vi "labHolo_path.vi"(2 "sub folder or file (path)  [ignored if str is not empty]":path, 3 "sub folder or file (str)":string) -> (0 "Exists?":bool, 1 "labHolo path":path)   [LabVIEW 2022 SP3]
panel:
  out "sub folder names":string[](array[string])
  out "sub filenames":string[](array[string])
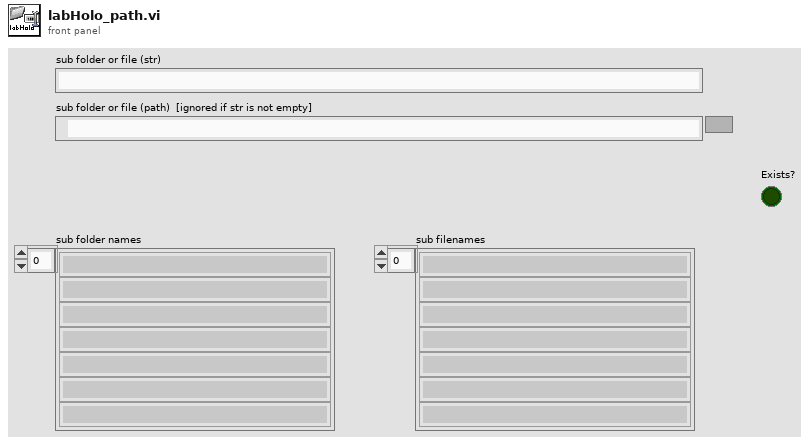
[diagram p1: front panel]
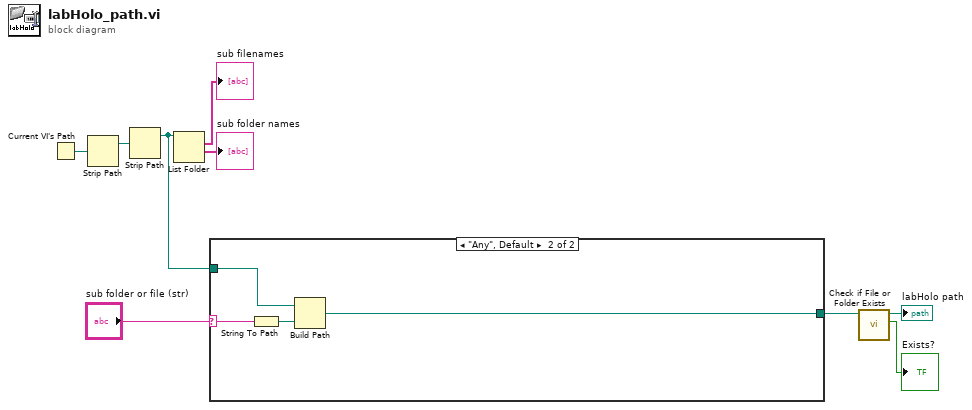
[diagram p0: block diagram]
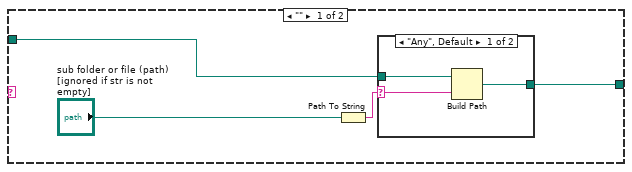
[diagram p2: hidden frame]
diagram:
  n1 = Current VI's Path() -> (path=w9:path)
  n2 = Strip Path(path=w9) -> (stripped path=w8:path)  [unwired: 1 out]
  n3 = Strip Path(path=w8) -> (stripped path=w4:path)  [unwired: 1 out]
  n4 = List Folder(path=w4) -> (filenames=→"sub filenames":string[], folder names=→"sub folder names":string[])  [unwired: 3 in, 2 out]
  n5 = case shown="\"Any\", Default" "sub folder or file (str)" {
    selector: "sub folder or file (str)" -> [_ w21]
    tunnel: w4 -> [w13 w19]
    tunnel: [w10 w20] -> w2
    frame "" {
      n6 = Path To String(path="sub folder or file (path)  [ignored if str is not empty]") -> (string=w11:string)
      n7 = case shown="\"Any\", Default" w11 {
        selector: w11 -> [w16 _]
        tunnel: w13 -> [w15 w17]
        tunnel: [w14 w17] -> w10
        frame "Any", Default {
          n8 = Build Path(base path=w15, name or relative path=w16) -> (appended path=w14:path)
        }
        frame "" {
        }
      }
    }
    frame "Any", Default {
      n9 = String To Path(string=w21) -> (path=w18:path)
      n10 = Build Path(base path=w19, name or relative path=w18) -> (appended path=w20:path)
    }
  }
  n11 = call <vilib>:"Check if File or Folder Exists.vi"("path"=w2) -> ("file or folder exists?"=→"Exists?":bool, "dup path"=→"labHolo path":path)  [unwired: 8 in, 1 out]
